vi "Einzel Range.vi"(2 "Inj image Readback":dbl, 3 "Inj image Einzel Set":dbl) -> (1 "Einzel  Range":bool)   [LabVIEW 2016, in "Low energy.lvlib"]
doc: "This takes the readback and setpoint for an Einzel lens and checks to see if\nit is within a certain range"
uses:
  Low energy.lvlib
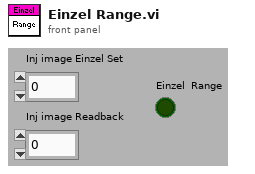
[diagram p1: front panel]
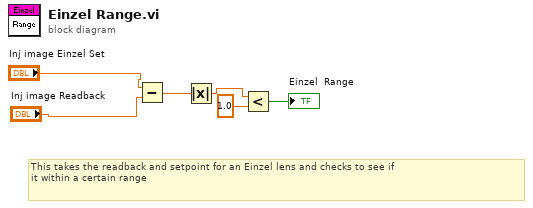
[diagram p0: block diagram]
diagram:
  # "This takes the readback and setpoint for an Einzel lens and checks to see if\nit within a certain range"
  n1 = Subtract(x="Inj image Einzel Set", y="Inj image Readback") -> (x-y=w4:dbl)
  n2 = Absolute Value(x=w4) -> (abs(x)=w3:dbl)
  n3 = Less?(x=w3, y=1.0) -> (x < y?=→"Einzel  Range":bool)
